vi "Write Teller.vi"(10 "Teller":T1 {"Absolute Time" format="%<%x %.3X>T"}, 11 "Stop Msg Input in":refnum<class "Stop Msg Input.lvclass">) -> (3 "Stop Msg Input out":refnum<class "Stop Msg Input.lvclass">)   [LabVIEW 2020, in "jettl.lvlib" / "Stop jettl Msg.lvlib" / "Stop Msg Input.lvlib" / "Stop Msg Input.lvclass"]
uses:
  Stop Msg Input.lvclass
  Teller Metadata/Teller Metadata.lvclass
  Stop Msg Input.lvclass/Stop Msg Input.ctl
  Relation.ctl
  jettl.lvlib
  Teller.ctl
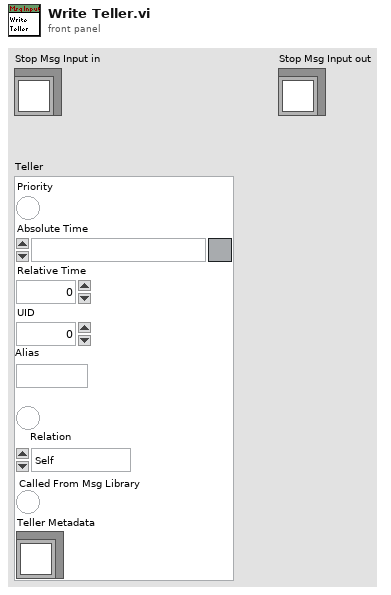
[diagram p1: front panel]
types:
  T1 = typedef "jettl.lvlib/Teller.ctl" = cluster{"Priority":bool, "Absolute Time":timestamp, "Relative Time":dbl, "UID":i32, "Alias":string, "Valid Relation":bool, "Relation":T2, "Called From Msg Library":bool, "Teller Metadata":refnum<class "Teller Metadata.lvclass">}
  T2 = typedef "jettl.lvlib/Relation.ctl" = enum16{"Self", "Parent", "Child"}
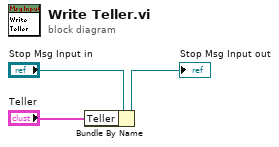
[diagram p0: block diagram]
diagram:
  n1 = Bundle By Name(cluster="Stop Msg Input in", "Teller"="Teller") -> (→"Stop Msg Input out":refnum<class "Stop Msg Input.lvclass">)
